vi "Byte generator.vi"() -> ()   [LabVIEW 2024]
panel:
  in  "RGBW Cluster":T1
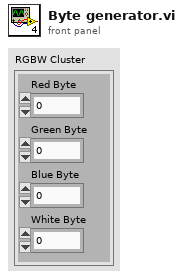
[diagram p1: front panel]
types:
  T1 = cluster{"Red Byte":u8, "Green Byte":u8, "Blue Byte":u8, "White Byte":u8}
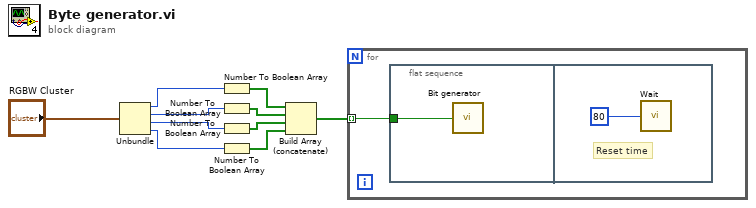
[diagram p0: block diagram]
diagram:
  n1 = Unbundle("RGBW Cluster") -> ("Red Byte"=w5:u8, "Green Byte"=w3:u8, "Blue Byte"=w2:u8, "White Byte"=w1:u8)
  n2 = Number To Boolean Array(number=w5) -> (Boolean array=w7:bool[])
  n3 = Number To Boolean Array(number=w3) -> (Boolean array=w10:bool[])
  n4 = Number To Boolean Array(number=w2) -> (Boolean array=w9:bool[])
  n5 = Number To Boolean Array(number=w1) -> (Boolean array=w8:bool[])
  n6 = Build Array (concatenate)(w7, w10, w9, w8) -> (w6:bool[])
  n7 = for {
    tunnel: w6 -> [w11] mode=indexing
    n8 = flat-sequence {
      tunnel: w11 -> [w12]
      frame #0 {
        n9 = call "Bit generator.vi"("Bit"=w12) -> ()
      }
      frame #1 {
        # "Reset time"
        n10 = call "Wait"("Count(uSec)"=u8 80) -> ()  [unwired: 1 out]
      }
    }
  }
